vi "FPGA_PPG_query_clock_rate.vi"(0 "resource_in":refnum<visa-resource-name>, 5 "error in (no error)":errorcluster) -> (14 "resource_out":refnum<visa-resource-name>, 16 "clockRate [ticks/us]":i32, 19 "error out":errorcluster)   [LabVIEW 2014, in "NI-FPGA_PPG_Driver.lvlib"]
doc: "Queries the clock-rate of the single-cycle-loop of the FPGA. The single-cycle-loop is responsible for producing the bit patterns by executing the commands that have been configured previously."
uses:
  NI-FPGA_PPG_Driver.lvlib
  FPGA_PPG_action_type.ctl
  <vilib>/Utility/error.llb/Error Cluster From Error Code.vi
  <vilib>/rvi/errors/niLvFpgaAdjustHostInterfaceError.vi
  <vilib>/rvi/interface/nirviReadWriteControl/nirviReadWriteControl.xnode
  FPGA_PPG_vi_ref.ctl
  FPGA Bitfiles/TiTaProj_COF_PPG_d3vptxinz-s.lvbitx
  NiFpgaLv.dll
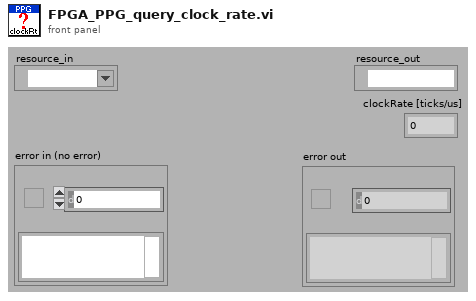
[diagram p1: front panel]
types:
  T1 = typedef "NI-FPGA_PPG_Driver.lvlib/FPGA_PPG_action_type.ctl" = enum16{"GET", "SET", "REMOVE"}
  T2 = typedef "NI-FPGA_PPG_Driver.lvlib/FPGA_PPG_vi_ref.ctl" = refnum<k20>
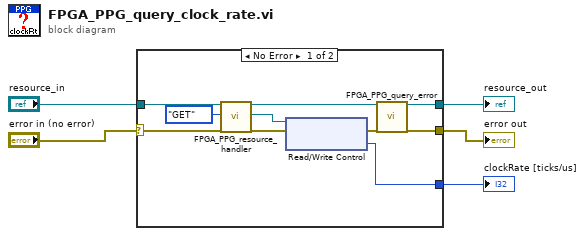
[diagram p0: block diagram]
diagram:
  n1 = case shown="No Error" "error in (no error)" {
    selector: "error in (no error)" -> [w14 w17]
    tunnel: [w8 w17] -> w4
    tunnel: [w11 w16] -> w3
    tunnel: "resource_in" -> [w15 w16]
    tunnel: [w12 _] -> w1
    frame No Error {
      n2 = call "FPGA_PPG_resource_handler.vi"("resource_in"=w15, "action"=FPGA_PPG_action_type."GET", "error in (no error)"=w14) -> ("resource_out"=w10:refnum<visa-resource-name>, "FPGA VI Reference Out"=w6:T2, "error out"=w13:errorcluster)  [unwired: 14 in]
      n3 = xnode "Read/Write Control"("FPGA VI Reference In"=w6, "error in"=w13) -> ("error out"=w9:errorcluster, "ticks_per_us"=w12:i32)  [unwired: 1 out]
      n4 = call "FPGA_PPG_query_error.vi"("resource_in"=w10, "error in (no error)"=w9) -> ("resource_out"=w11:refnum<visa-resource-name>, "error out"=w8:errorcluster)  [unwired: 16 in]
    }
    frame Error {
    }
  }
  "error out" <- w4
  "resource_out" <- w3
  "clockRate [ticks/us]" <- w1
